vi "Global Variables.vi"() -> ()   [LabVIEW 2013, in "VirtualRobot.lvlib"]
uses:
  VirtualRobot.lvlib
  <vilib>/ActorFramework/Message Enqueuer/Message Enqueuer.lvclass
panel:
  out "DriveTrain":refnum<class "Message Enqueuer.lvclass">
  out "Driver":refnum<class "Message Enqueuer.lvclass">
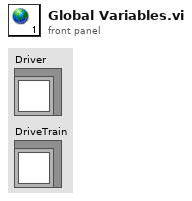
[diagram p1: front panel]
diagram:
